vi "Get Most Recent Color Image16.vi"(6 "blue":u16, 7 "green":u16, 9 "red":u16, 10 "algorithm":i32, 11 "size":u32) -> (1 "red out":u16, 3 "function return":u32, 4 "blue out":u16, 5 "green out":u16)   [LabVIEW 2018, in "Copy of Andor SDK.lvlib"]
doc: "EXPNETTYPE unsigned int WINAPI GetMostRecentColorImage16(unsigned long size, int algorithm, WORD * red, WORD * green, WORD * blue);"
uses:
  Copy of Andor SDK.lvlib
  <userlib>/Andor SDK/ATMCD32D.dll
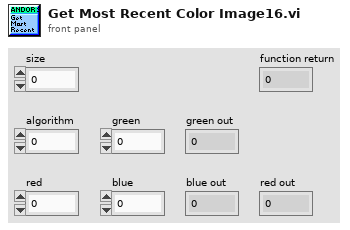
[diagram p1: front panel]
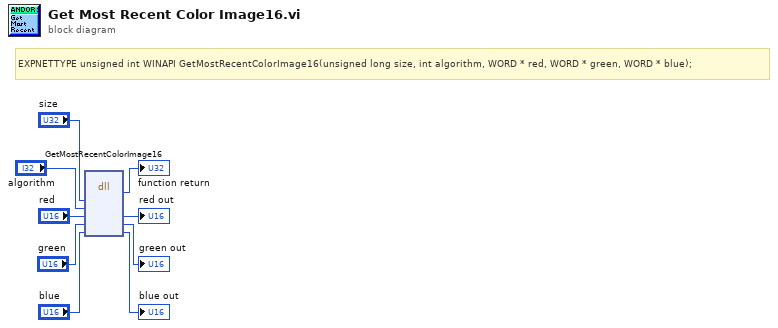
[diagram p0: block diagram]
diagram:
  # "EXPNETTYPE unsigned int WINAPI GetMostRecentColorImage16(unsigned long size, int algorithm, WORD * red, WORD * green, WORD * blue);"
  n1 = dll-call lib="C:/Program Files (x86)/National Instruments/LabVIEW 2018/user.lib/Andor SDK/ATMCD32D.*" fn="GetMostRecentColorImage16"("size"="size", "algorithm"="algorithm", "red"="red", "green"="green", "blue"="blue") -> (→"function return":u32, "red"=→"red out":u16, "green"=→"green out":u16, "blue"=→"blue out":u16)  [unwired: 5 in, 2 out]
